vi "save.vi"(8 "error in (no error)":errorcluster, 9 "base name":string, 10 "folder path":path, 11 "DL090215DataCollection in":refnum<class "DataCollectionDL091104Scaffold.lvclass">) -> (0 "error out":errorcluster, 3 "DL090215DataCollection out":refnum<class "DataCollectionDL091104Scaffold.lvclass">)   [LabVIEW 2010, in "DataCollectionDL091104Scaffold.lvclass"]
uses:
  DataCollectionDL091104Scaffold.lvclass
  common/classes/ErrorController/ErrorController/class_data.vi
  common/classes/NoteBook/Notebook/Notebook.lvclass
  common/classes/ErrorController/ErrorController/ErrorController.lvclass
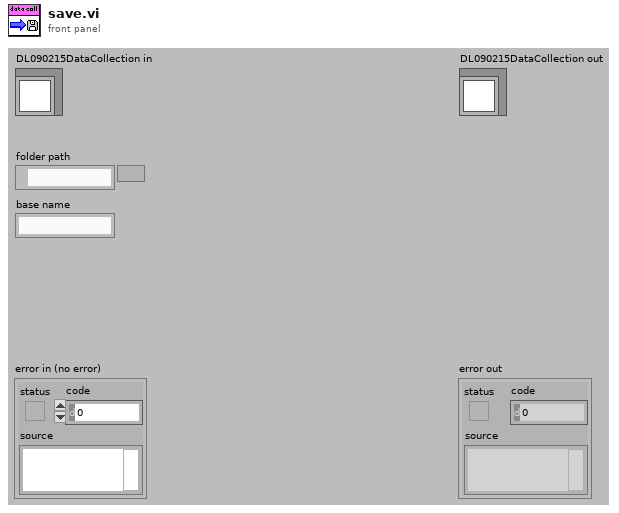
[diagram p1: front panel]
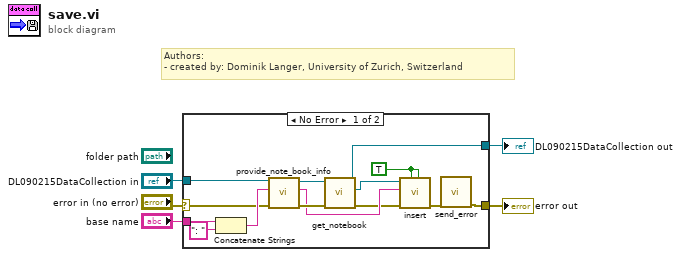
[diagram p0: block diagram]
diagram:
  # "Authors: \n- created by: Dominik Langer, University of Zurich, Switzerland"
  n1 = case shown="No Error" "error in (no error)" {
    selector: "error in (no error)" -> [w11 w21]
    tunnel: [w12 w21] -> w4
    tunnel: [w15 w20] -> w2
    tunnel: "DL090215DataCollection in" -> [w10 w20]
    tunnel: "base name" -> [w13 _]
    frame No Error {
      w6 = TRUE ("add line break before?")
      n2 = Concatenate Strings(w13, ": " ("string")) -> (w16:string)
      n3 = call-dynamic "provide_note_book_info.vi"("error in (no error)"=w11, "notebook string in"=w16, "DataCollectionDL091104Scaffold in"=w10) -> ("error out"=w19:errorcluster, "notebook string out"=w17:string, "DataCollectionDL091104Scaffold out"=w18:refnum<class "DataCollectionDL091104Scaffold.lvclass">)  [unwired: 6 in]
      n4 = call-dynamic "get_notebook.vi"("error in (no error)"=w19, "GenericComponent in"=w18) -> ("error out"=w8:errorcluster, "notebook"=w9:refnum<class "Notebook.lvclass">, "GenericComponent out"=w15:refnum<class "DataCollectionDL091104Scaffold.lvclass">)  [unwired: 7 in]
      n5 = call "insert.vi"("add line break after?"=w6, "add line break before?"=w6, "error in (no error)"=w8, "string"=w17, "Notebook in"=w9) -> ("error out"=w7:errorcluster)  [unwired: 6 out]
      n6 = call "send_error.vi"("error in (no error)"=w7) -> ("error out"=w12:errorcluster)  [unwired: 10 in]
    }
    frame Error {
    }
  }
  "error out" <- w4
  "DL090215DataCollection out" <- w2
